vi "Write EvtParams.vi"(8 "error in (no error)":errorcluster, 10 "EvtParams":dbl[][](array[numeric]), 11 "VisualizeAppRingdown in":refnum<class "VisualizeAppRingdown.lvclass">) -> (0 "error out":errorcluster, 3 "VisualizeAppRingdown out":refnum<class "VisualizeAppRingdown.lvclass">)   [LabVIEW 2017, in "Visualization.lvlib" / "VisualizeAppRingdown.lvclass"]
uses:
  VisualizeAppRingdown.lvclass
  VisualizeAppRingdown.lvclass/VisualizeAppRingdown.ctl
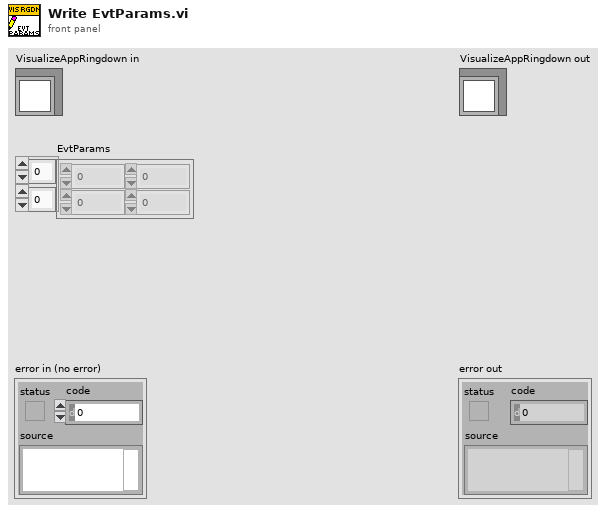
[diagram p1: front panel]
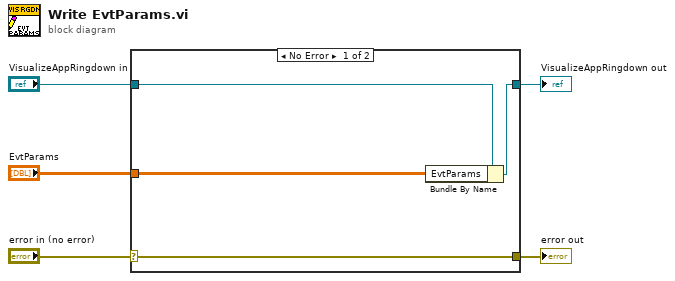
[diagram p0: block diagram]
diagram:
  n1 = case shown="No Error" "error in (no error)" {
    selector: "error in (no error)" -> [w9 w10]
    tunnel: [w9 w10] -> w4
    tunnel: [w7 w11] -> w2
    tunnel: "VisualizeAppRingdown in" -> [w8 w11]
    tunnel: "EvtParams" -> [w6 _]
    frame No Error {
      n2 = Bundle By Name(cluster=w8, "EvtParams"=w6) -> (w7:refnum<class "VisualizeAppRingdown.lvclass">)
    }
    frame Error {
    }
  }
  "error out" <- w4
  "VisualizeAppRingdown out" <- w2
